vi "unpackLocalPara.vi"(6 "长度":i32, 7 "数据":u8[](array[numeric]) format="%.0x") -> (2 "输出通道":u8, 3 "本机表参数":cluster{"有功常数":i32, "无功常数":i32, "输出类型":i32})   [LabVIEW 2014]
panel:
  out "告警信息":string
  # "默认0"
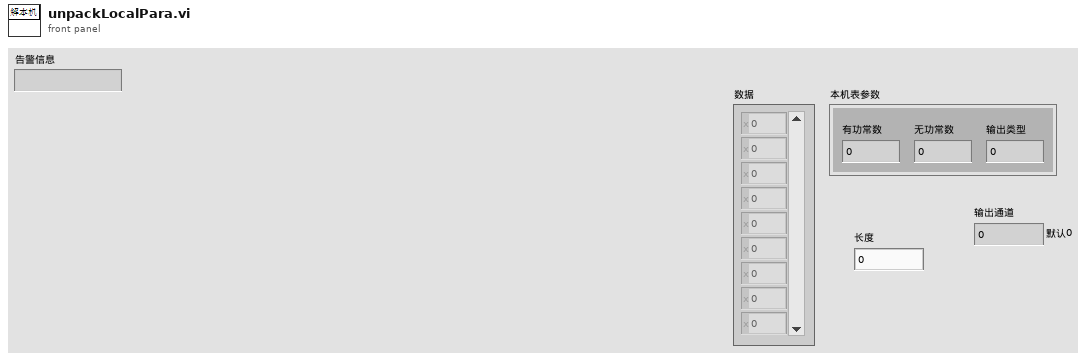
[diagram p1: front panel]
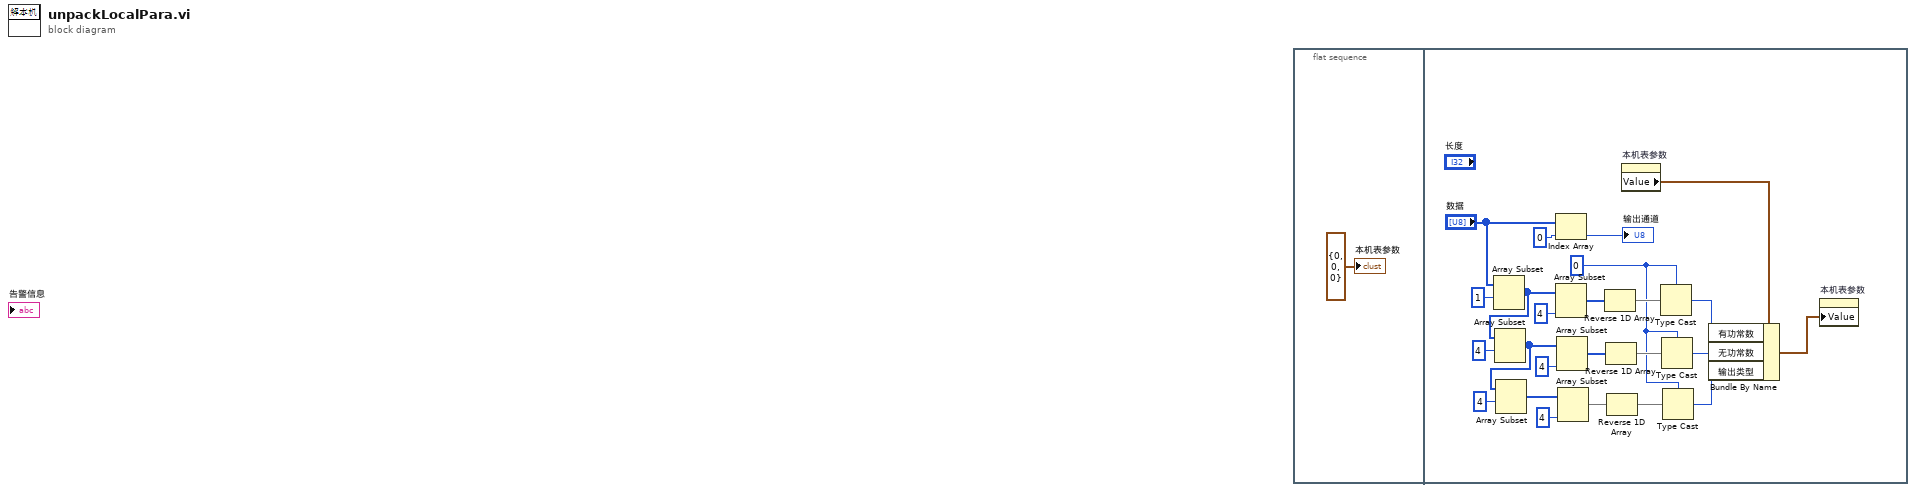
[diagram p0: block diagram]
diagram:
  n1 = flat-sequence {
    frame #0 {
      "本机表参数" <- cluster{"有功常数":i32, "无功常数":i32, "输出类型":i32} {"有功常数"=0, "无功常数"=0, "输出类型"=0} ("本机表参数")
    }
    frame #1 {
      w7 = 0
      n2 = Array Subset(array="数据", index=1 ("索引")) -> (w9:u8[])  [unwired: 1 in]
      n3 = Array Subset(array=w9, index=4 ("索引")) -> (w8:u8[])  [unwired: 1 in]
      n4 = Array Subset(array=w8, index=4 ("索引")) -> (w12:u8[])  [unwired: 1 in]
      n5 = Index Array(array="数据", index=0 ("索引")) -> (element=→"输出通道":u8)
      n6 = Array Subset(array=w9, length=4 ("长度")) -> (w20:u8[])  [unwired: 1 in]
      n7 = Array Subset(array=w8, length=4 ("长度")) -> (w17:u8[])  [unwired: 1 in]
      n8 = Array Subset(array=w12, length=4 ("长度")) -> (w11:u8[])  [unwired: 1 in]
      n9 = Reverse 1D Array(array=w20) -> (reversed array=w19:u8[])
      n10 = Reverse 1D Array(array=w17) -> (reversed array=w18:u8[])
      n11 = Reverse 1D Array(array=w11) -> (reversed array=w10:u8[])
      n12 = property on="本机表参数" class="Clust (严格)"() -> ("Value"=w5:cluster{"有功常数":i32, "无功常数":i32, "输出类型":i32})  [unwired: 2 in, 2 out]
      n13 = Type Cast(type=w7, x=w19) -> (*(type *) &x=w3:i32)
      n14 = Type Cast(type=w7, x=w18) -> (*(type *) &x=w6:i32)
      n15 = Type Cast(type=w7, x=w10) -> (*(type *) &x=w4:i32)
      n16 = Bundle By Name(cluster=w5, "有功常数"=w3, "无功常数"=w6, "输出类型"=w4) -> (w2:cluster{"有功常数":i32, "无功常数":i32, "输出类型":i32})
      n17 = property on="本机表参数" class="Clust (严格)"("Value"=w2) -> ()  [unwired: 2 in, 2 out]
    }
  }
